vi "Destroy.vi"(8 "Error In":errorcluster, 11 "reference in":refnum<class "OD Sub-Entry.lvclass">) -> (0 "Error Out":errorcluster, 3 "reference out":refnum<class "OD Sub-Entry.lvclass">)   [LabVIEW 2019, in "Electronic Datasheet.lvlib" / "OD Sub-Entry.lvclass"]
uses:
  OD Sub-Entry.lvclass
  OD Entry/OD Entry.lvclass
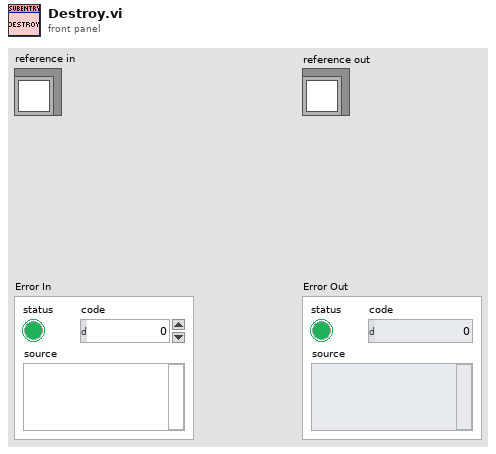
[diagram p1: front panel]
types:
  T1 = typedef "Electronic Datasheet.lvlib/OD Sub-Entry.lvclass/ObjectAttributes.ctl" = cluster{"Parent":refnum<class "OD Entry.lvclass">}
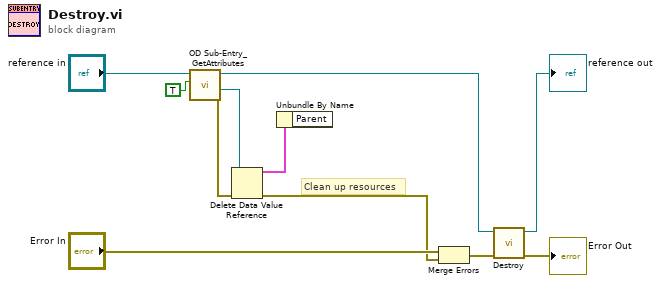
[diagram p0: block diagram]
diagram:
  # "Clean up resources"
  n1 = call "OD Sub-Entry_GetAttributes.vi"("OnlyGetDvrReference(False)"=TRUE, "reference in"="reference in") -> ("Error Out"=w10:errorcluster, "DataRef"=w9:refnum<data-value>, "reference out"=w2:refnum<class "OD Sub-Entry.lvclass">)  [unwired: 6 in, 1 out]
  n2 = Delete Data Value Reference(data value reference=w9, error in=w10) -> (data value=w4:T1, error out=w7:errorcluster)
  n3 = Unbundle By Name(w4) -> ()  [unwired: 1 out]
  n4 = Merge Errors("Error In", w7) -> (w11:errorcluster)
  n5 = call-parent "Destroy.vi"("Error In"=w11, "reference in"=w2) -> ("Error Out"=→"Error Out":errorcluster, "reference out"=→"reference out":refnum<class "OD Sub-Entry.lvclass">)  [unwired: 8 in]
